vi "Read Publish Msg.vi"(11 "IModel in":refnum<class "IModel.lvclass">) -> (2 "Pre-Addressed Publish Msg":refnum<class "Publish Msg.lvclass">, 3 "IModel out":refnum<class "IModel.lvclass">)   [LabVIEW 2015, in "IModel.lvlib" / "IModel.lvclass"]
uses:
  IModel.lvclass
  IMediator/IMediator Messages/Publish Msg/Publish Msg.lvclass
  IModel.lvclass/IModel.ctl
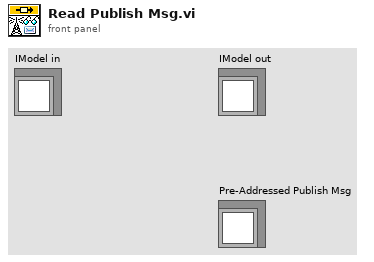
[diagram p1: front panel]
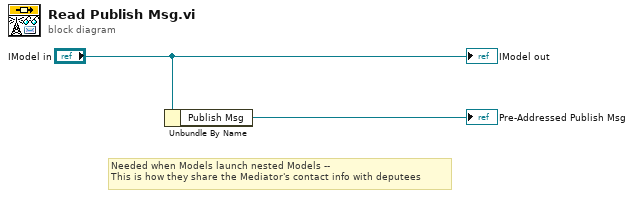
[diagram p0: block diagram]
diagram:
  # "Needed when Models launch nested Models --\nThis is how they share the Mediator's contact info with deputees"
  n1 = Unbundle By Name("IModel in") -> ("Publish Msg"=→"Pre-Addressed Publish Msg":refnum<class "Publish Msg.lvclass">)
  "IModel out" <- "IModel in"
